vi "Open VI Reference.vi"(7 "password":string, 8 "error in":errorcluster, 9 "options":i32, 10 "VI Path":string) -> (0 "error out":errorcluster, 3 "VI Refnum":refnum<vi>)   [LabVIEW 2026, in "G-AI Core.lvlib"]
doc: "Wrapper for \"Open VI Reference\" function. Use this instead of the original function to make sure the VI Reference stays alive even if the tool finishes execution.\n\n_____\nCreated using DQMH Framework: Event Scripter 7.1.2.1547."
uses:
  G-AI Core.lvlib
  Open VI Reference Argument--cluster.ctl
  Open VI Reference (Reply Payload)--cluster.ctl
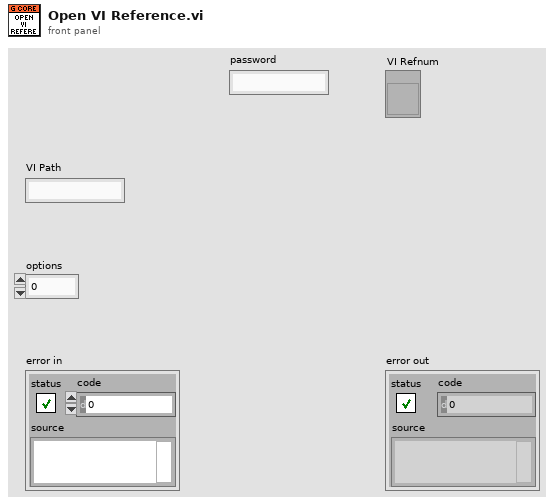
[diagram p1: front panel]
types:
  T1 = typedef "G-AI Core.lvlib/Open VI Reference Argument--cluster.ctl" = cluster{"VI Path":string, "options":i32, "password":string, "Wait Notifier":refnum<notifier>, "wait for reply":bool}
  T2 = typedef "G-AI Core.lvlib/Request Events--cluster.ctl" = cluster{"Stop Module":refnum<user-event>, "Show Panel":refnum<user-event>, "Hide Panel":refnum<user-event>, "Get Module Execution Status":refnum<user-event>, "Show Diagram":refnum<user-event>, "Store Reference":refnum<user-event>, "Get Reference":refnum<user-event>, "New VI":refnum<user-event>, "Open VI Reference":refnum<user-event>}
  T3 = typedef "G-AI Core.lvlib/Open VI Reference (Reply Payload)--cluster.ctl" = cluster{"VI Refnum":refnum<vi>, "error":errorcluster}
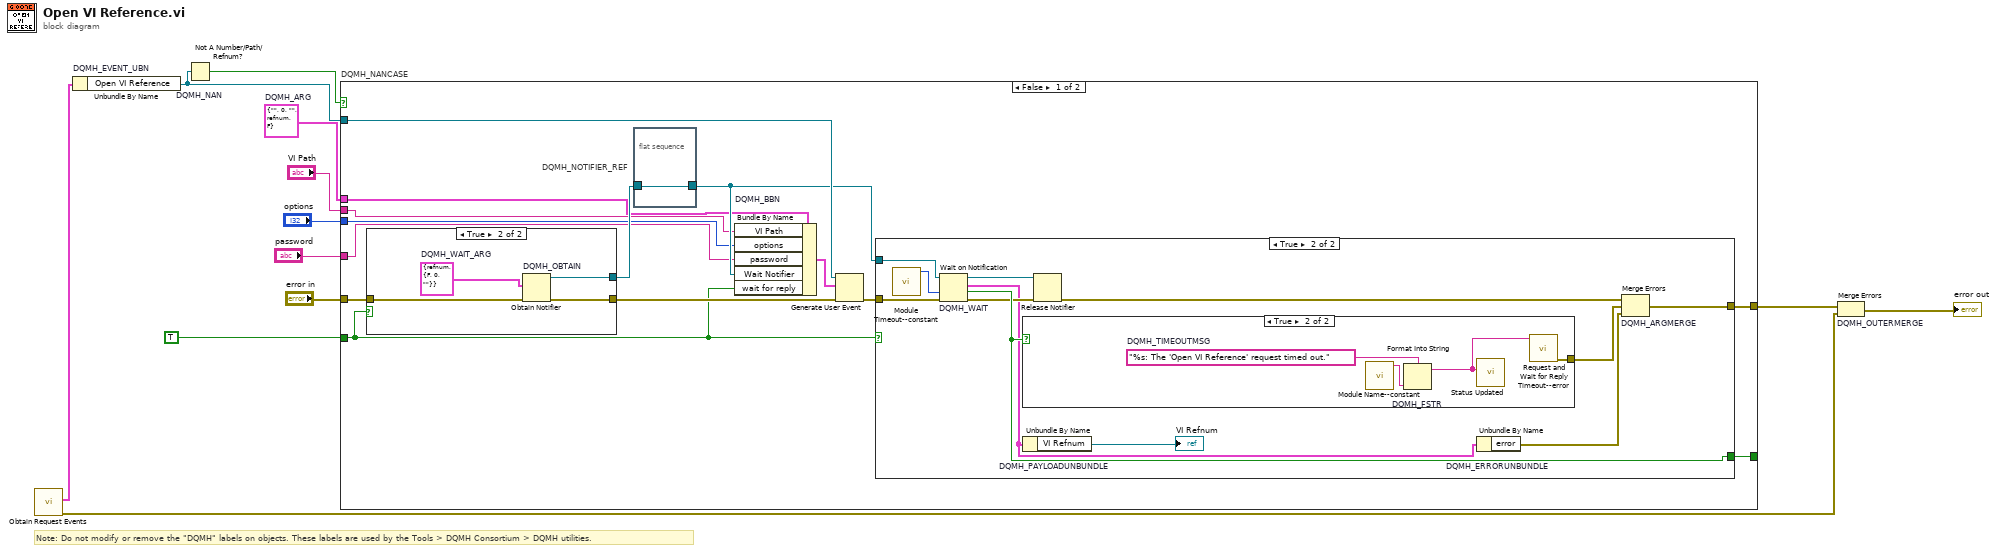
[diagram p0: block diagram]
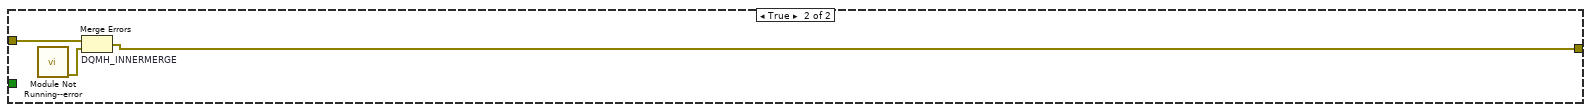
[diagram p5: hidden frame]
diagram:
  w7 = T1 {"VI Path"="", "options"=0, "password"="", "Wait Notifier"=refnum, "wait for reply"=FALSE}  # DQMH_ARG
  # "Note: Do not modify or remove the \"DQMH\" labels on objects. These labels are used by the Tools > DQMH Consortium > DQMH utilities."
  n1 = call "Obtain Request Events.vi"() -> ("error out"=w2:errorcluster, "G-AI Core Request Events"=w1:T2)  [unwired: 10 in]
  n2 = Unbundle By Name "DQMH_EVENT_UBN"(w1) -> ("Open VI Reference"=w10:refnum<user-event>)
  n3 = Not A Number/Path/Refnum? "DQMH_NAN"(number/path/refnum=w10) -> (NaN/Path/Refnum?=w9:bool)
  n4 = case "DQMH_NANCASE" shown="False" w9 {
    tunnel: "error in" -> [w26 w52]
    tunnel: w10 -> [w24 _]
    tunnel: [w21 w51] -> w8
    tunnel: [w22 _] -> _
    tunnel: w7 -> [w17 _]
    tunnel: "VI Path" -> [w16 _]
    tunnel: "options" -> [w15 _]
    tunnel: "password" -> [w14 _]
    tunnel: TRUE ("wait for reply (T)") -> [w13 _]
    frame False {
      n5 = case shown="True" w13 {
        tunnel: w26 -> [w45 w49]
        tunnel: [w45 w48] -> w23
        tunnel: [_ w46] -> w19
        frame False {
        }
        frame True {
          w47 = T3 {"VI Refnum"=refnum, "error"={"status"=FALSE, "code"=0, "source"=""}}  # DQMH_WAIT_ARG
          n6 = Obtain Notifier "DQMH_OBTAIN"(notification data type=w47, error in (no error)=w49) -> (notifier out=w46:refnum<notifier>, error out=w48:errorcluster)  [unwired: 2 in, 1 out]
        }
      }
      n7 = flat-sequence "DQMH_NOTIFIER_REF" {
        tunnel: w19 -> [w27]
        tunnel: [w27] -> w18
        frame #0 {
        }
      }
      n8 = Bundle By Name "DQMH_BBN"(cluster=w17, "VI Path"=w16, "options"=w15, "password"=w14, "Wait Notifier"=w18, "wait for reply"=w13) -> (w20:T1)
      n9 = Generate User Event(user event=w24, event data cluster=w20, error in=w23) -> (error out=w25:errorcluster)  [unwired: 1 in, 1 out]
      n10 = case shown="True" w13 {
        tunnel: w25 -> [w28 w40]
        tunnel: w18 -> [_ w39]
        tunnel: [_ w37] -> w22
        tunnel: [w28 w36] -> w21
        frame False {
        }
        frame True {
          n11 = call "Module Timeout--constant.vi"() -> ("Module Timeout"=w30:i32)  [unwired: 11 in]
          n12 = Wait on Notification "DQMH_WAIT"(notifier=w39, timeout in ms (-1)=w30, error in (no error)=w40) -> (notifier out=w38:refnum<notifier>, notification=w31:T3, timed out?=w37:bool, error out=w35:errorcluster)  [unwired: 1 in]
          n13 = case shown="True" w37 {
            tunnel: [_ w42] -> w32
            frame False {
            }
            frame True {
              w44 = "%s: The 'Open VI Reference' request timed out."  # DQMH_TIMEOUTMSG
              n14 = call "Module Name--constant.vi"() -> ("Module Name"=w41:string)  [unwired: 11 in]
              n15 = Format Into String "DQMH_FSTR"(format string=w44, w41) -> (resulting string=w43:string)  [unwired: 2 in, 1 out]
              n16 = call "Status Updated.vi"("Status"=w43) -> ()  [unwired: 10 in, 1 out]
              n17 = call "Request and Wait for Reply Timeout--error.vi"("Error Message"=w43) -> ("error out"=w42:errorcluster)  [unwired: 10 in]
            }
          }
          n18 = Unbundle By Name "DQMH_PAYLOADUNBUNDLE"(w31) -> ("VI Refnum"=→"VI Refnum":refnum<vi>)
          n19 = Release Notifier(notifier=w38, error in (no error)=w35) -> (error out=w34:errorcluster)  [unwired: 1 in, 2 out]
          n20 = Unbundle By Name "DQMH_ERRORUNBUNDLE"(w31) -> ("error"=w33:errorcluster)
          n21 = Merge Errors "DQMH_ARGMERGE"(w34, w32, w33) -> (w36:errorcluster)
        }
      }
    }
    frame True {
      n22 = call "Module Not Running--error.vi"() -> ("error out"=w50:errorcluster)  [unwired: 11 in]
      n23 = Merge Errors "DQMH_INNERMERGE"(w52, w50) -> (w51:errorcluster)
    }
  }
  n24 = Merge Errors "DQMH_OUTERMERGE"(w8, w2) -> (→"error out":errorcluster)
